vi "Main Action Process Loop.vi"(8 "error in (no error)":errorcluster, 11 "Main Process Class In":refnum<class "Main Class.lvclass">) -> ()   [LabVIEW 2019]
uses:
  Class/Main Process Class/Main Class.lvclass
  Class/Main Process Class/MPC_AutoPaste/Ctrl/123.ctl
  Control Loop/Ctrl/Control Loop_Control.ctl
  Control Loop/Ctrl/Control Loop_Status.ctl
  Class/Main Process Class/MPC_AutoPaste/Global/Process Global.vi
  LLB/Commonly VI/Main Glb.vi
  LLB/Commonly VI.lvlib
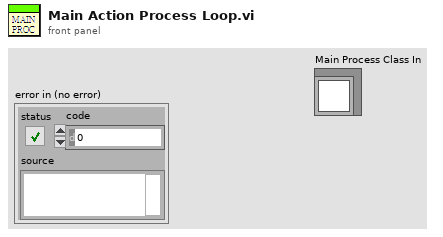
[diagram p1: front panel]
types:
  T1 = enum16{"Initial", "Add", "Read", "Delete & Check"}
  T2 = typedef "123.ctl" = enum16{"Initial", "Write", "Read"}
  T3 = typedef "Control Loop_Control.ctl" = enum16{"Initial", "Standby Mode", "Run Mode", "Status", "Exit"}
  T4 = typedef "Control Loop_Status.ctl" = enum16{"None", "Next", "Error", "SafeDoor", "Exit"}
  T5 = cluster{"Control":T3, "Status":T4, "Name":string, "error":errorcluster}
  T6 = cluster{"AutoRunFlg":refnum<vi>, "Action Finish Flg":refnum<vi>, "Remaining Action":refnum<vi>, "Btn_AutoRun":refnum<vi>, "Manual Flg":refnum<vi>, "Sub Process Error":refnum<vi>}
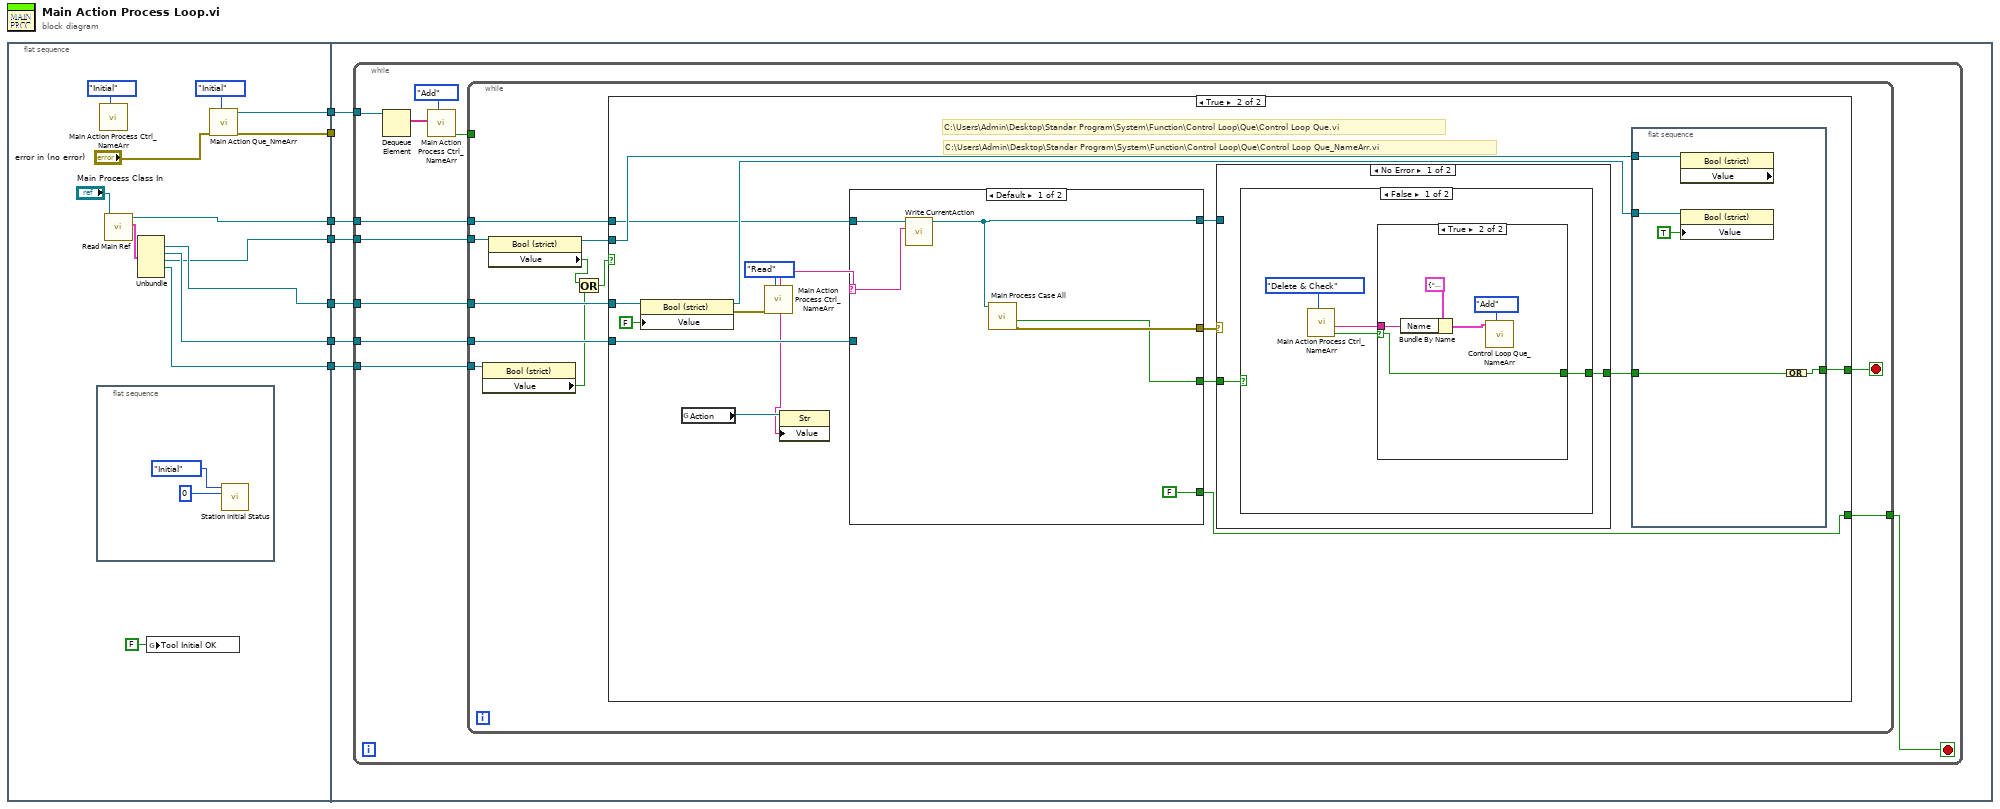
[diagram p0: block diagram]
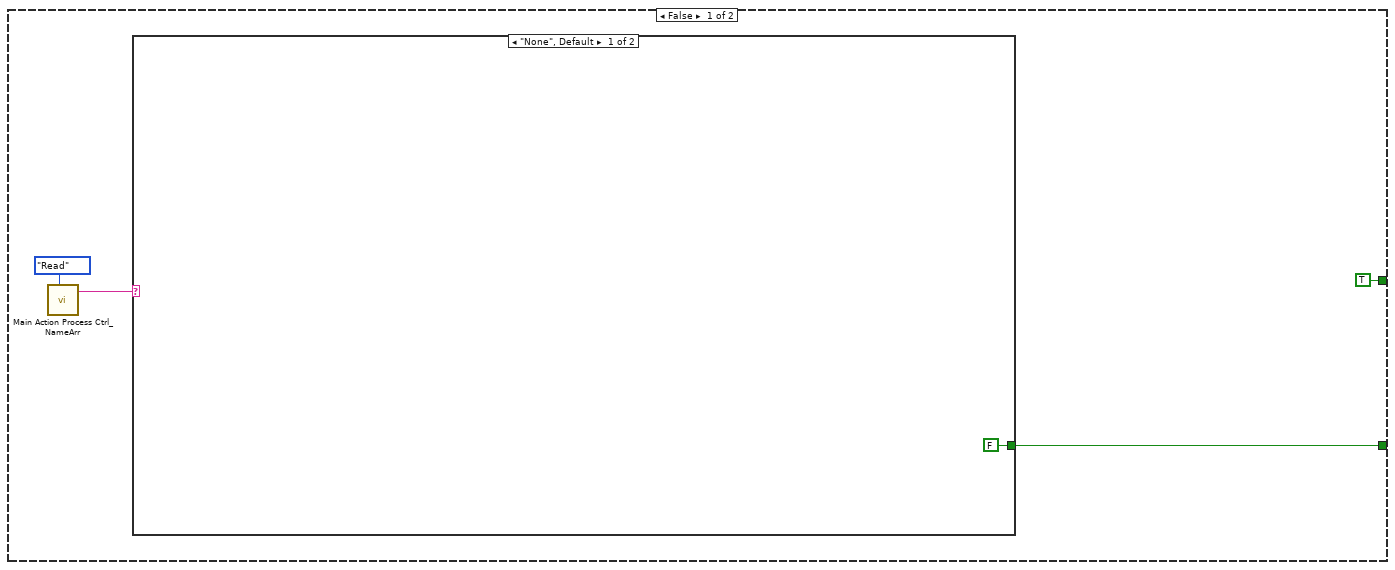
[diagram p2: hidden frame]
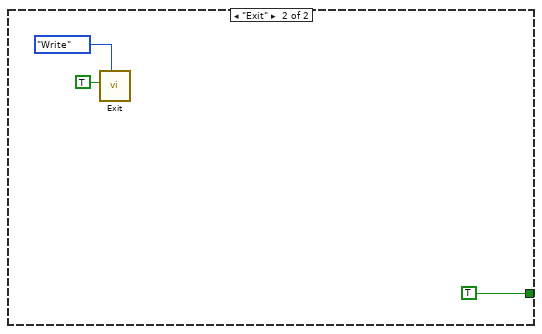
[diagram p3: hidden frame]
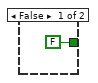
[diagram p4: hidden frame]
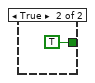
[diagram p5: hidden frame]
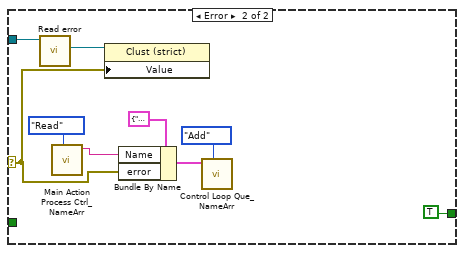
[diagram p6: hidden frame]
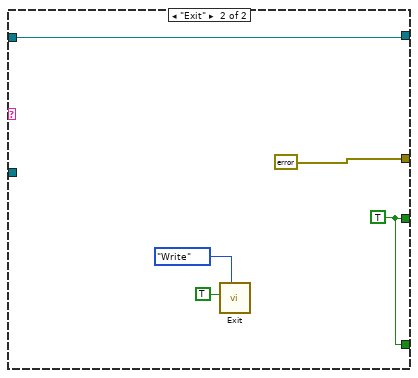
[diagram p7: hidden frame]
diagram:
  n1 = flat-sequence {
    tunnel: [w18] -> w7
    tunnel: [w17] -> w6
    tunnel: [w9] -> w5
    tunnel: [w15] -> w4
    tunnel: [w14] -> w3
    tunnel: [w12] -> w2
    tunnel: [w10] -> w1
    tunnel: w7 -> [_]
    tunnel: w6 -> [w28]
    tunnel: w5 -> [w27]
    tunnel: w4 -> [w26]
    tunnel: w3 -> [w25]
    tunnel: w2 -> [w24]
    tunnel: w1 -> [w23]
    frame #0 {
      n2 = flat-sequence {
        frame #0 {
          n3 = call "Station Initial Status.vi"("Insert"=0, "Enum"=123."Initial") -> ()  [unwired: 8 in, 2 out]
        }
      }
      n4 = call "Main Action Process Ctrl_NameArr.vi"("Action"=T1."Initial") -> ()  [unwired: 6 in, 5 out]
      n5 = call-dynamic "Read Main Ref.vi"("Main Process Class in"="Main Process Class In") -> ("Main Ref"=w11:T6, "Main Process Class out"=w12:refnum<class "Main Class.lvclass">)  [unwired: 8 in, 1 out]
      n6 = Unbundle(w11) -> ("Action Finish Flg"=w15:refnum<vi>, "Remaining Action"=w14:refnum<vi>, "Btn_AutoRun"=w9:refnum<vi>, "Manual Flg"=w10:refnum<vi>)  [unwired: 2 out]
      n7 = global write "Process Global.vi" "Tool Initial OK"(FALSE ("Tool Initial OK")) -> ()
      n8 = call "Main Action Que_NmeArr.vi"("Action"=enum16{"Initial", "Add", "Release"}."Initial", "error in (no error)"="error in (no error)") -> ("error out"=w18:errorcluster, "Process Que Out"=w17:refnum<queue>)  [unwired: 8 in]
    }
    frame #1 {
      n9 = while {
        tunnel: w28 -> [w38]
        tunnel: w27 -> [w35]
        tunnel: w26 -> [w34]
        tunnel: w25 -> [w31]
        tunnel: w24 -> [w30]
        tunnel: w23 -> [w29]
        stop <- w33 stop-if-true
        n10 = Dequeue Element(queue=w38) -> (element=w32:string[])  [unwired: 2 in, 3 out]
        n11 = call "Main Action Process Ctrl_NameArr.vi"("Action"=T1."Add", "Add Action Que"=w32) -> ("Finish"=w36:bool)  [unwired: 5 in, 4 out]
        n12 = while {
          tunnel: w36 -> [_]
          tunnel: w35 -> [w49]
          tunnel: w34 -> [w48]
          tunnel: [w45] -> w33
          tunnel: w31 -> [w40]
          tunnel: w30 -> [w44]
          tunnel: w29 -> [w41]
          stop <- w46 stop-if-true
          n13 = property class="Bool (strict)"(reference=w41) -> ("Value"=w39:bool)  [unwired: 1 in, 2 out]
          n14 = property class="Bool (strict)"(reference=w49) -> (reference out=w47:refnum<vi>, "Value"=w43:bool)  [unwired: 1 in, 1 out]
          n15 = Or(x=w43, y=w39) -> (x .or. y?=w42:bool)
          n16 = case shown="True" w42 {
            tunnel: w48 -> [_ w72]
            tunnel: w47 -> [_ w65]
            tunnel: [TRUE w64] -> w46
            tunnel: [w52 w61] -> w45
            tunnel: w40 -> [_ w63]
            tunnel: w44 -> [_ w62]
            frame False {
              n17 = call "Main Action Process Ctrl_NameArr.vi"("Action"=T1."Read") -> ("Read Action"=w50:string)  [unwired: 6 in, 4 out]
              n18 = case shown="\"None\", Default" w50 {
                tunnel: [FALSE TRUE] -> w52
                frame "None", Default {
                }
                frame "Exit" {
                  n19 = call "Exit.vi"("Enum"=enum16{"Initial", "Read", "Write"}."Write", "ExitIn"=TRUE) -> ()  [unwired: 9 in, 1 out]
                }
              }
            }
            frame True {
              # "C:\\Users\\Admin\\Desktop\\Standar Program\\System\\Function\\Control Loop\\Que\\Control Loop Que_NameArr.vi"
              # "C:\\Users\\Admin\\Desktop\\Standar Program\\System\\Function\\Control Loop\\Que\\Control Loop Que.vi"
              n20 = property class="Bool (strict)"(reference=w72, "Value"=FALSE) -> (reference out=w67:refnum<vi>, error out=w70:errorcluster)  [unwired: 1 in]
              n21 = global read "Main Glb.vi" "Action"() -> (w59:refnum<vi>)
              n22 = call "Main Action Process Ctrl_NameArr.vi"("Action"=T1."Read", "error in"=w70) -> ("Read Action"=w58:string)  [unwired: 5 in, 4 out]
              n23 = property class="Str"(reference=w59, "Value"=w58) -> ()  [unwired: 1 in, 2 out]
              n24 = case shown="Default" w58 {
                selector: w58 -> [w103 _]
                tunnel: [w105 errorcluster {"status"=FALSE, "code"=0, "source"=""} ("error constant")] -> w69
                tunnel: [w104 w110] -> w68
                tunnel: w62 -> [w106 w107]
                tunnel: w63 -> [_ _]
                tunnel: [FALSE w110] -> w61
                tunnel: [w101 w107] -> w60
                frame Default {
                  n25 = call-dynamic "Write CurrentAction.vi"("CurrentAction"=w103, "Main Process Class in"=w106) -> ("Main Process Class out"=w101:refnum<class "Main Class.lvclass">)  [unwired: 8 in, 1 out]
                  n26 = call "Main Process Case All.vi"("Main Process Class In"=w101) -> ("error out"=w105:errorcluster, "KeepCase"=w104:bool)  [unwired: 9 in]
                }
                frame "Exit" {
                  w110 = TRUE
                  n27 = call "Exit.vi"("Enum"=enum16{"Initial", "Read", "Write"}."Write", "ExitIn"=TRUE) -> ()  [unwired: 9 in, 1 out]
                }
              }
              n28 = case shown="No Error" w69 {
                selector: w69 -> [_ w92]
                tunnel: w68 -> [w80 _]
                tunnel: [w79 TRUE] -> w66
                tunnel: w60 -> [_ w94]
                frame No Error {
                  n29 = case shown="False" w80 {
                    tunnel: [w82 TRUE] -> w79
                    frame False {
                      n30 = call "Main Action Process Ctrl_NameArr.vi"("Action"=T1."Delete & Check") -> ("Finish"=w83:bool, "Delete Action"=w81:string)  [unwired: 6 in, 3 out]
                      n31 = case shown="True" w83 {
                        selector: w83 -> [_ w88]
                        tunnel: w81 -> [_ w89]
                        tunnel: [FALSE w88] -> w82
                        frame False {
                        }
                        frame True {
                          n32 = Bundle By Name(cluster=T5 {"Control"=enum."Status", "Status"=enum."Next", "Name"="", "error"={"status"=FALSE, "code"=0, "source"=""}} ("Control Loop In"), "Name"=w89) -> (w86:T5)
                          n33 = call "Control Loop Que_NameArr.vi"("Action Select"=enum16{"Initial", "Add", "Release"}."Add", "Control Loop In"=w86) -> ()  [unwired: 8 in, 2 out]
                        }
                      }
                    }
                    frame True {
                    }
                  }
                }
                frame Error {
                  n34 = call-dynamic "Read error.vi"("Main Class in"=w94) -> ("error"=w93:refnum<vi>)  [unwired: 8 in, 2 out]
                  n35 = call "Main Action Process Ctrl_NameArr.vi"("Action"=T1."Read") -> ("Read Action"=w97:string)  [unwired: 6 in, 4 out]
                  n36 = property class="Clust (strict)"(reference=w93, "Value"=w92) -> ()  [unwired: 1 in, 2 out]
                  n37 = Bundle By Name(cluster=T5 {"Control"=enum."Status", "Status"=enum."Error", "Name"="", "error"={"status"=FALSE, "code"=0, "source"=""}} ("Control Loop In"), "Name"=w97, "error"=w92) -> (w95:T5)
                  n38 = call "Control Loop Que_NameArr.vi"("Action Select"=enum16{"Initial", "Add", "Release"}."Add", "Control Loop In"=w95) -> ()  [unwired: 8 in, 2 out]
                }
              }
              n39 = flat-sequence {
                tunnel: w67 -> [w78]
                tunnel: w66 -> [w75]
                tunnel: w65 -> [w76]
                tunnel: [w74] -> w64
                frame #0 {
                  n40 = property class="Bool (strict)" props=["Value"](reference=w76) -> ()  [unwired: 1 in, 3 out]
                  n41 = property class="Bool (strict)"(reference=w78, "Value"=TRUE) -> ()  [unwired: 1 in, 2 out]
                  n42 = Compound Arithmetic op=OR(w75) -> (w74:bool)
                }
              }
            }
          }
        }
      }
    }
  }
